vi "R_생성시퀀스.vi"(8 "error in":errorcluster, 10 "Result data":T1={"NG OK"=TRUE, "Data int"=0, "Daa dbl"=0.0, "Result"=""}) -> (0 "error out":errorcluster)   [LabVIEW 2019]
uses:
  _ctrl/create-rw-close.ctl
  _ctrl/rw.ctl
  _ctrl/BP4610_cmd.ctl
  _ctrl/DSP_action.ctl
  _ctrl/start.ctl
  <vilib>/DAQmx/create/channels.llb/DAQmx Create Channel (DO-Digital Output).vi
  <vilib>/DAQmx/write.llb/DAQmx Write (Digital Bool 1Line 1Point).vi
  state-machine_result.ctl
panel:
  in  "sequence":string
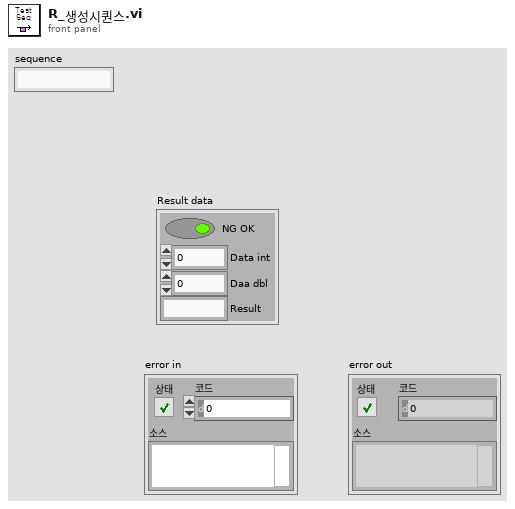
[diagram p1: front panel]
types:
  T1 = typedef "state-machine_result.ctl" = cluster{"NG OK":bool, "Data int":i32, "Daa dbl":dbl, "Result":string}
  T2 = typedef "rw.ctl" = enum16{"read", "write"}
  T3 = typedef "BP4610_cmd.ctl" = enum16{"open", "read", "set", "limit", "output", "close"}
  T4 = typedef "create-rw-close.ctl" = enum16{"create", "write", "read", "close"}
  T5 = typedef "BP4610_cmd.ctl" = enum16{"open", "read", "set", "limit", "output on", "output off", "close"}
  T6 = typedef "DSP_action.ctl" = enum16{"False", "cont", "on", "off", "discont", "protection", "preread", "level", "read", "stop", "exit"}
  T7 = typedef "DSP_action.ctl" = enum16{"False", "cont", "on", "off", "discont", "apply", "preread", "level", "read", "stop", "exit"}
  T8 = typedef "start.ctl" = enum16{"init", "open", "set", "start", "stop", "read", "read_items", "query", "close", "T_single", "reset", "exit"}
  T9 = typedef "Tap_내구시험.ctl" = enum32{"특성시험", "그래프", "환경설정", "장비"}
  T10 = enum8{"Enabled", "Disabled", "Disabled and Grayed Out"}
  T11 = cluster{"시작":refnum<vi>, "RESET":refnum<vi>, "정지":refnum<vi>, "Exit":refnum<vi>, "대기":refnum<vi>, "Main":refnum<vi>, "시험세팅":refnum<vi>, "그래프":refnum<vi>}
  T12 = typedef "Testing-info.ctl" = cluster{"전체채널수":u8, "현재채널번호":u8, "Irms":dbl, "입력전압":dbl, "입력전류":dbl, "출력전압":dbl, "출력전류":dbl, "온도":dbl, "제어단 단선":bool, "제어단 단락":bool, "제어단 특성변화":bool, "출력단 단선":bool, "출력단 단락":bool, "출력단 특성변화":bool, "출력단 전압":bool, "카운트 일치":bool, "Irms 판정":bool, "온도":bool, "테스트 회수":u32}
  T13 = cluster{"Relay 1":refnum<vi>, "Relay 2":refnum<vi>, "Relay 3":refnum<vi>, "Relay 4":refnum<vi>, "Relay 5":refnum<vi>, "Relay 6":refnum<vi>, "고장진단 기준 값":refnum<vi>, "wfm 1":refnum<vi>, "wfm 3":refnum<vi>, "wfm 2":refnum<vi>, "wfm 4":refnum<vi>, "wfm 5":refnum<vi>, "wfm 6":refnum<vi>, "Tab Control":refnum<vi>}
  T14 = typedef "DL950_wfms.ctl" = cluster{"wfms":waveform(dbl)[], "Waveform_2":cluster{"t0":dbl, "dt":dbl, "Y":dbl[][]}, "items":dbl[][]}
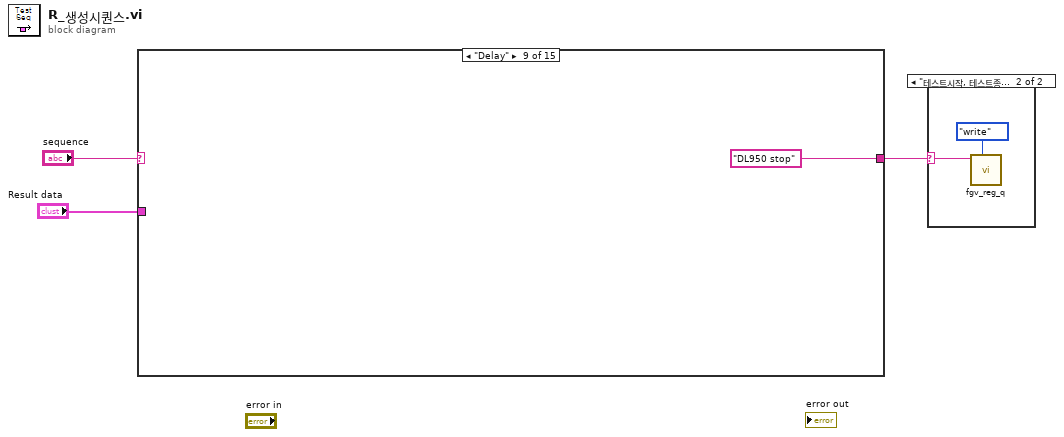
[diagram p0: block diagram]
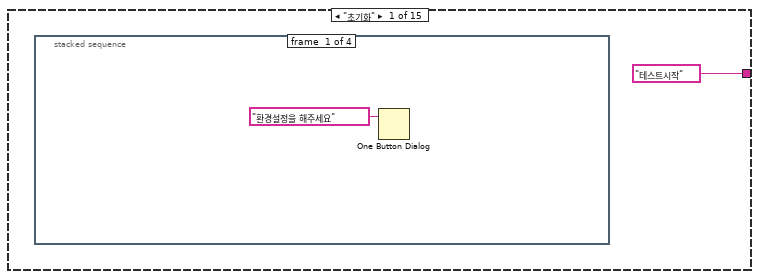
[diagram p3: hidden frame]
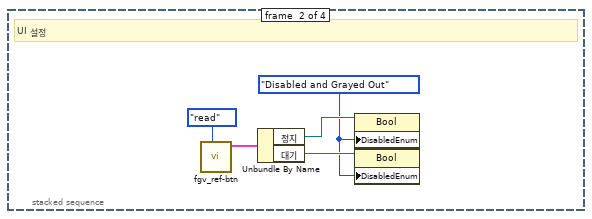
[diagram p4: hidden frame]
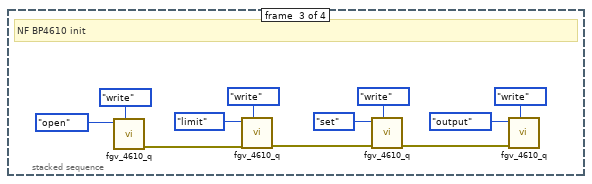
[diagram p5: hidden frame]
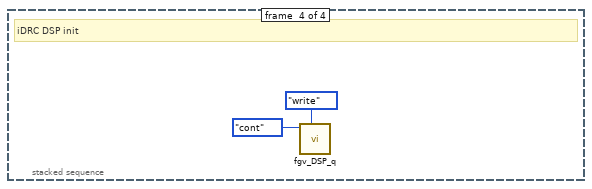
[diagram p6: hidden frame]
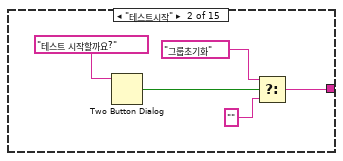
[diagram p7: hidden frame]
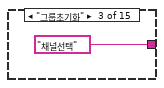
[diagram p8: hidden frame]
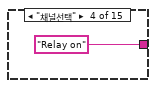
[diagram p9: hidden frame]
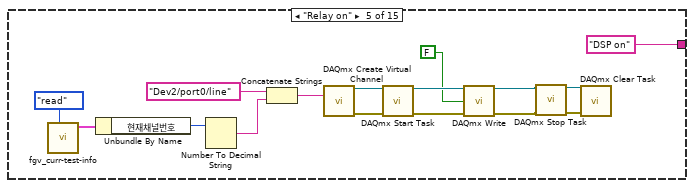
[diagram p10: hidden frame]
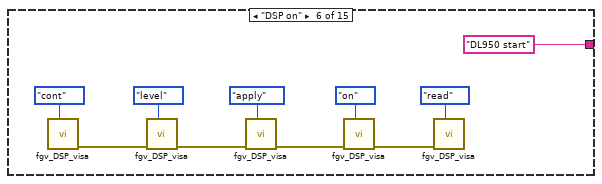
[diagram p11: hidden frame]
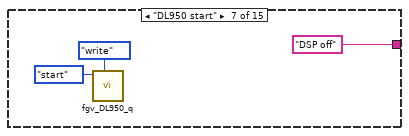
[diagram p12: hidden frame]
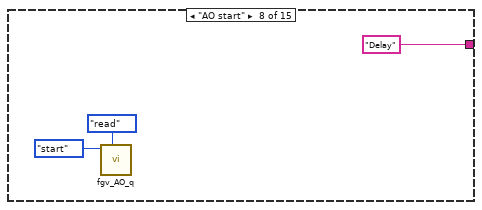
[diagram p13: hidden frame]
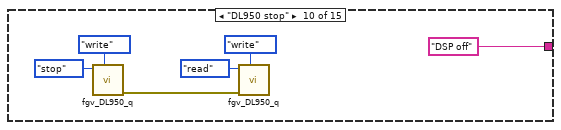
[diagram p14: hidden frame]
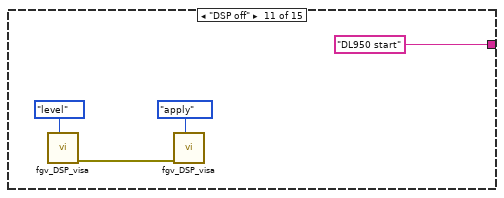
[diagram p15: hidden frame]
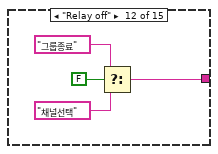
[diagram p16: hidden frame]
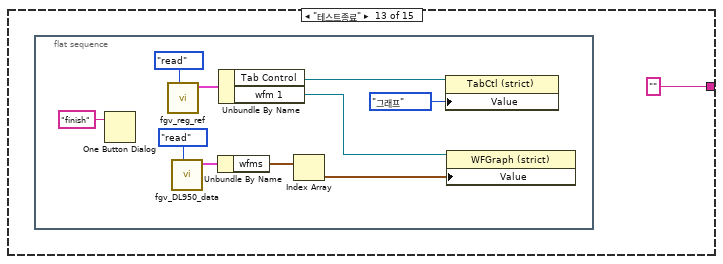
[diagram p17: hidden frame]
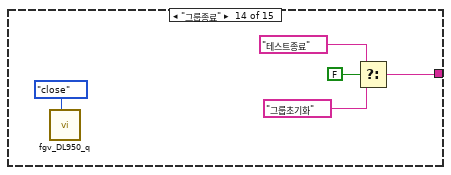
[diagram p18: hidden frame]
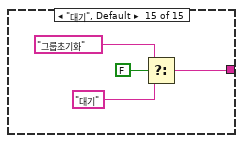
[diagram p19: hidden frame]
diagram:
  n1 = case shown="\"Delay\"" "sequence" {
    tunnel: ["테스트시작" w24 "채널선택" "Relay on" "DSP on" "DL950 start" "DSP off" "Delay" "DL950 stop" "DSP off" "DL950 start" w75 "" w91 w97] -> w3
    tunnel: "Result data" -> [_ _ _ _ _ _ _ _ _ _ _ _ _ _ _]
    frame "초기화" {
      n2 = stacked-sequence {
        frame #0 {
          n3 = One Button Dialog(message="환경설정을 해주세요" ("메시지")) -> ()  [unwired: 1 in, 1 out]
        }
        frame #1 {
          w7 = T10."Disabled and Grayed Out" ("비활성화")
          # "UI 설정"
          n4 = call "fgv_ref-btn.vi"("cmd"=rw."read") -> ("ref 2"=w10:T11)  [unwired: 10 in]
          n5 = Unbundle By Name(w10) -> ("정지"=w9:refnum<vi>, "대기"=w8:refnum<vi>)
          n6 = property class="Bool"(reference=w9, "DisabledEnum"=w7) -> ()  [unwired: 1 in, 2 out]
          n7 = property class="Bool"(reference=w8, "DisabledEnum"=w7) -> ()  [unwired: 1 in, 2 out]
        }
        frame #2 {
          # "NF BP4610 init"
          n8 = call "fgv_4610_q.vi"("cmd"=create-rw-close."write", "action"=BP4610_cmd."open") -> ("error out"=w17:errorcluster)  [unwired: 8 in, 1 out]
          n9 = call "fgv_4610_q.vi"("cmd"=create-rw-close."write", "error in"=w17, "action"=BP4610_cmd."limit") -> ("error out"=w12:errorcluster)  [unwired: 7 in, 1 out]
          n10 = call "fgv_4610_q.vi"("cmd"=create-rw-close."write", "error in"=w12, "action"=BP4610_cmd."set") -> ("error out"=w11:errorcluster)  [unwired: 7 in, 1 out]
          n11 = call "fgv_4610_q.vi"("cmd"=create-rw-close."write", "error in"=w11, "action"=BP4610_cmd."output") -> ()  [unwired: 7 in, 2 out]
        }
        frame #3 {
          # "iDRC DSP init"
          n12 = call "fgv_DSP_q.vi"("cmd"=create-rw-close."write", "action"=DSP_action."cont") -> ()  [unwired: 8 in, 2 out]
        }
      }
    }
    frame "테스트시작" {
      n13 = Two Button Dialog(message="테스트 시작할까요?" ("메시지")) -> (T button?=w27:bool)  [unwired: 2 in]
      n14 = Select(t="그룹초기화", s=w27, f="") -> (s? t:f=w24:string)
    }
    frame "그룹초기화" {
    }
    frame "채널선택" {
    }
    frame "Relay on" {
      n15 = call "fgv_curr-test-info.vi"("cmd"=rw."read") -> ("현재테스트 정보 2"=w44:T12)  [unwired: 10 in]
      n16 = Unbundle By Name(w44) -> ("현재채널번호"=w32:u8)
      n17 = Number To Decimal String(number=w32) -> (decimal integer string=w31:string)  [unwired: 1 in]
      n18 = Concatenate Strings("Dev2/port0/line", w31) -> (w33:string)
      n19 = call-poly <vilib>:"DAQmx Create Virtual Channel.vi"("lines"=w33) -> ("task out"=w37:refnum<k21>, "error out"=w36:errorcluster)  [unwired: 13 in]
      n20 = call <vilib>:"DAQmx Start Task.vi"("task/channels in"=w37, "error in"=w36) -> ("task out"=w40:refnum<k21>, "error out"=w41:errorcluster)  [unwired: 12 in]
      n21 = call-poly <vilib>:"DAQmx Write.vi"("task/channels in"=w40, "data"=FALSE, "error in"=w41) -> ("task out"=w42:refnum<k21>, "error out"=w43:errorcluster)  [unwired: 10 in, 1 out]
      n22 = call <vilib>:"DAQmx Stop Task.vi"("task/channels in"=w42, "error in"=w43) -> ("task out"=w38:refnum<k21>, "error out"=w39:errorcluster)  [unwired: 12 in]
      n23 = call <vilib>:"DAQmx Clear Task.vi"("task in"=w38, "error in"=w39) -> ()  [unwired: 13 in, 1 out]
    }
    frame "DSP on" {
      n24 = call "fgv_DSP_visa.vi"("action"=DSP_action."cont") -> ("error out"=w51:errorcluster)  [unwired: 10 in]
      n25 = call "fgv_DSP_visa.vi"("action"=DSP_action."level", "error in"=w51) -> ("error out"=w50:errorcluster)  [unwired: 9 in]
      n26 = call "fgv_DSP_visa.vi"("action"=DSP_action."apply", "error in"=w50) -> ("error out"=w49:errorcluster)  [unwired: 9 in]
      n27 = call "fgv_DSP_visa.vi"("action"=DSP_action."on", "error in"=w49) -> ("error out"=w47:errorcluster)  [unwired: 9 in]
      n28 = call "fgv_DSP_visa.vi"("action"=DSP_action."read", "error in"=w47) -> ()  [unwired: 9 in, 1 out]
    }
    frame "DL950 start" {
      n29 = call "fgv_DL950_q.vi"("cmd"=create-rw-close."write", "data"=start."start") -> ()  [unwired: 8 in, 2 out]
    }
    frame "AO start" {
      n30 = call "fgv_AO_q.vi"("cmd"=create-rw-close."read", "data"=start."start") -> ()  [unwired: 8 in, 2 out]
    }
    frame "Delay" {
    }
    frame "DL950 stop" {
      n31 = call "fgv_DL950_q.vi"("cmd"=create-rw-close."write", "data"=start."stop") -> ("error out"=w64:errorcluster)  [unwired: 8 in, 1 out]
      n32 = call "fgv_DL950_q.vi"("cmd"=create-rw-close."write", "error in"=w64, "data"=start."read") -> ()  [unwired: 7 in, 2 out]
    }
    frame "DSP off" {
      n33 = call "fgv_DSP_visa.vi"("action"=DSP_action."level") -> ("error out"=w70:errorcluster)  [unwired: 10 in]
      n34 = call "fgv_DSP_visa.vi"("action"=DSP_action."apply", "error in"=w70) -> ()  [unwired: 9 in, 1 out]
    }
    frame "Relay off" {
      n35 = Select(t="그룹종료", s=FALSE, f="채널선택") -> (s? t:f=w75:string)
    }
    frame "테스트종료" {
      n36 = flat-sequence {
        frame #0 {
          n37 = One Button Dialog(message="finish" ("메시지")) -> ()  [unwired: 1 in, 1 out]
          n38 = call "fgv_reg_ref.vi"("cmd"=rw."read") -> ("output cluster 2"=w83:T13)  [unwired: 10 in]
          n39 = call "fgv_DL950_data.vi"("cmd"=rw."read") -> ("DL950 wfm 2"=w86:T14)  [unwired: 9 in, 1 out]
          n40 = Unbundle By Name(w86) -> ("wfms"=w87:waveform(dbl)[])
          n41 = Unbundle By Name(w83) -> ("Tab Control"=w84:refnum<vi>, "wfm 1"=w85:refnum<vi>)
          n42 = Index Array(array=w87) -> (element=w88:waveform(dbl))  [unwired: 1 in]
          n43 = property class="TabCtl (strict)"(reference=w84, "Value"=Tap_내구시험."그래프" ("값")) -> ()  [unwired: 1 in, 2 out]
          n44 = property class="WFGraph (strict)"(reference=w85, "Value"=w88) -> ()  [unwired: 1 in, 2 out]
        }
      }
    }
    frame "그룹종료" {
      n45 = call "fgv_DL950_q.vi"("cmd"=create-rw-close."close") -> ()  [unwired: 9 in, 2 out]
      n46 = Select(t="테스트종료", s=FALSE, f="그룹초기화") -> (s? t:f=w91:string)
    }
    frame "대기", Default {
      n47 = Select(t="그룹초기화", s=FALSE, f="대기") -> (s? t:f=w97:string)
    }
  }
  n48 = case shown="\"테스트시작, 테스트종료\", Default" w3 {
    selector: w3 -> [_ w98]
    frame "" {
    }
    frame "테스트시작, 테스트종료", Default {
      n49 = call "fgv_reg_q.vi"("cmd"=create-rw-close."write", "action"=w98) -> ()  [unwired: 8 in, 2 out]
    }
  }
